vi "PROJECTE OCELL FINAL 0.3.vi"() -> ()   [LabVIEW 2020]
uses:
  <vilib>/numeric/Random Number (Range) DBL.vi
  <vilib>/MakerHub/LINX/Public/Utilities/Open Serial.vi
  <vilib>/MakerHub/LINX/LMH-LINX.lvlib
  <vilib>/MakerHub/LINX/Public/Sensors/Distance/Ultrasonic/Ultrasonic.lvlib
panel:
  in  "DO Channel 2":u8=11
  in  "DI Channel 2":u8=10
  out "Error Out 2":errorcluster
  in  "Sensibilitat 2":dbl=10.0
  in  "Sensibilitat 1":dbl=10.0
  in  "DO Channel 1":u8=6
  out "?":string="HEU GUANYAT !!!"
  in  "TEMPS D'ESPERA":i32=30
  in  "Velocitat de moviment":u32=100
  out "Error Out 1":errorcluster
  in  "?":bool
  in  "DI Channel 1":u8=5
  out "Device Name":string
  in  "Error In":errorcluster
  in  "Baud Rate Override":u32=9600
  in  "Serial Port":refnum<visa-resource-name>="COM3"
  out "JOC COL·LABORATIU: encertar l'ocell":cluster{dbl[], dbl[]}[](graph)=[{[0.99, 0.985, 0.98, 0.975, 0.86, 0.88, 0.9, 0.92, 0.94, 0.96, 0.98, 1.0, 0.94, 0.96, 0.98, 0.86], [41.0, 42.0, 43.0, 44.0, 45.0, 45.0, 45.0, 45.0, 45.0, 45.0, 45.0, 45.0, 44.0, 43.0, 42.0, 45.5]}, {[0.0, 0.0, 0.0, 0.02, 0.02, 0.02, 0.04, 0.04, 0.06, -0.06, -0.04, -0.04, -0.02, -0.02, -0.02], [43.0, 45.0, 44.0, 45.0, 46.0, 44.0, 46.0, 47.0, 47.0, 47.0, 47.0, 46.0, 46.0, 44.0, 45.0]}, {[-0.99, -0.985, -0.98, -0.975, -0.86, -0.88, -0.9, -0.92, -0.94, -0.96, -0.98, -1.0, -0.94, -0.96, -0.98, -0.86], [41.0, 42.0, 43.0, 44.0, 45.0, 45.0, 45.0, 45.0, 45.0, 45.0, 45.0, 45.0, 44.0, 43.0, 42.0, 45.5]}]
  # "CONTROLS\nARDUINO"
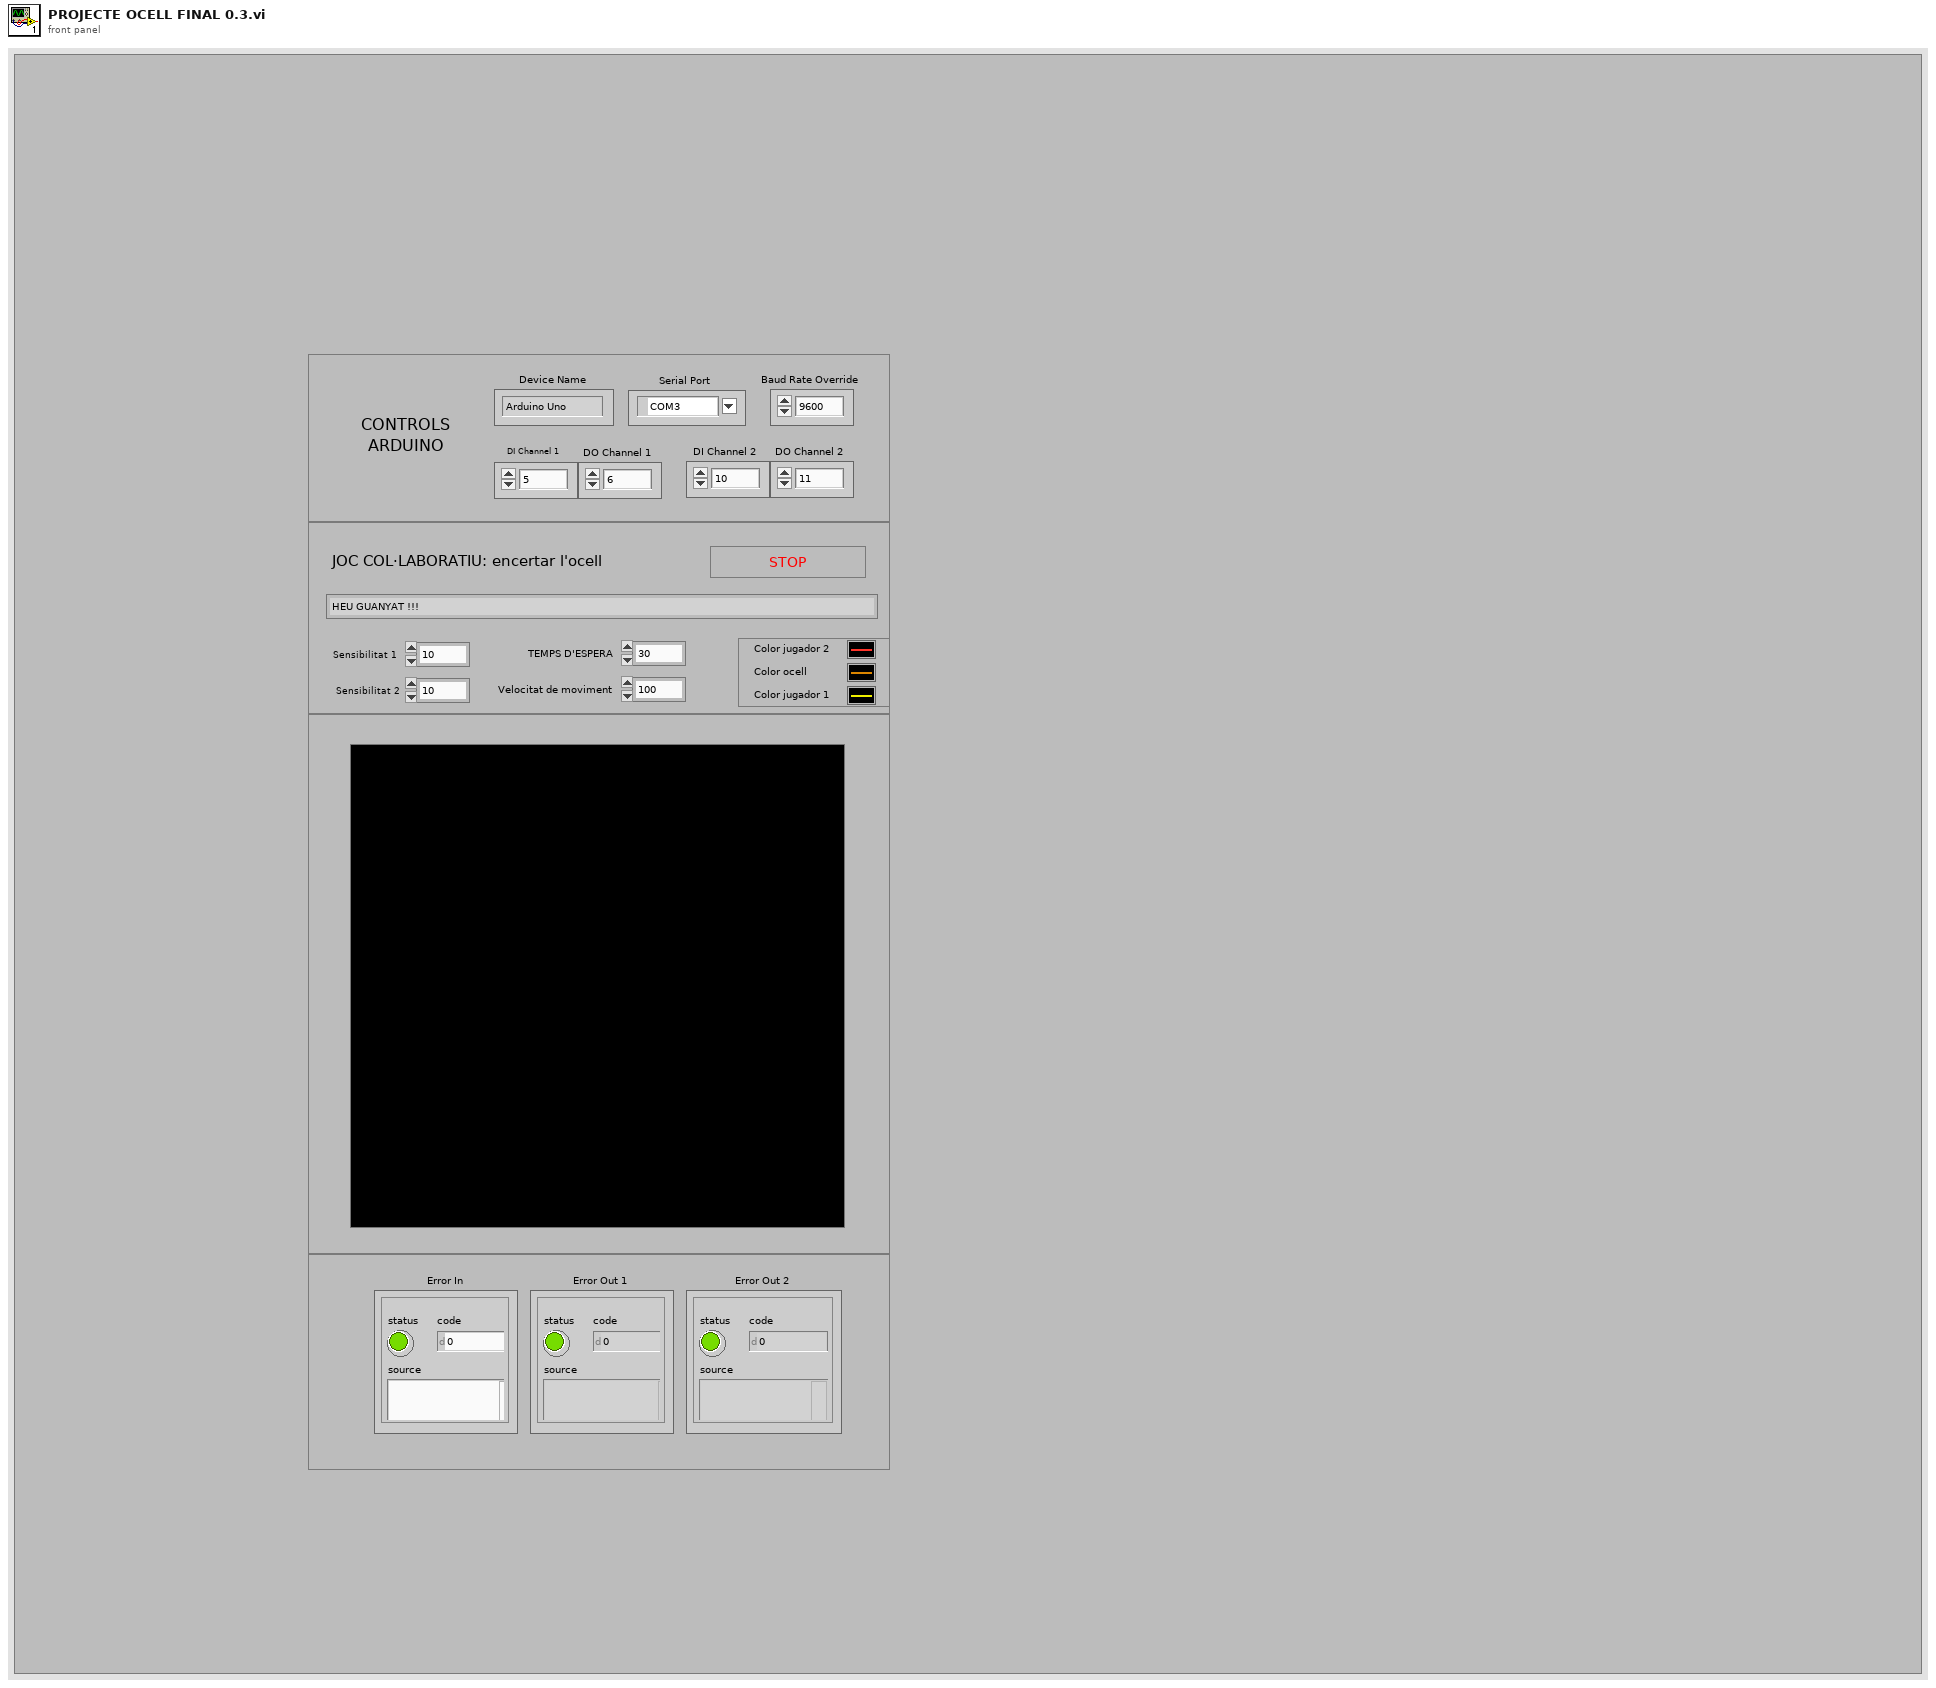
[diagram p1: front panel]
types:
  T1 = typedef "LMH-LINX.lvlib/LINX Ref.ctl" = cluster{"IO":T2, "Interface":T3, "LINX Device Config":T4}
  T2 = typedef "LMH-LINX.lvlib/Platform.ctl" = enum16{"Remote", "Local"}
  T3 = typedef "LMH-LINX.lvlib/Interface.ctl" = enum16{"Serial", "TCP"}
  T4 = typedef "LMH-LINX.lvlib/Device.lvlib/LINX Device Config.ctl" = cluster{"Interface":T3, "COM Port":refnum<visa-resource-name>, "TCP Configuration":T5, "Device Family":u8, "Device ID":u8, "Device Name":string, "TCP Ref":refnum<k5>, "Channels":T6}
  T5 = typedef "LMH-LINX.lvlib/Device.lvlib/TCP Config.ctl" = cluster{"IP Address":string, "Port":u16}
  T6 = typedef "LMH-LINX.lvlib/Channels.ctl" = cluster{"DI":u8[], "DO":u8[], "AI":u8[], "AO":u8[], "PWM":u8[], "QE":u8[], "UART":u8[], "I2C 2":u8[], "SPI":u8[], "CAN":u8[], "Servo":u8[], "AI Ref (V)":dbl, "AI Resolution (Bits)":u8, "AO Ref (V)":dbl, "AO Resolution (Bits)":u8}
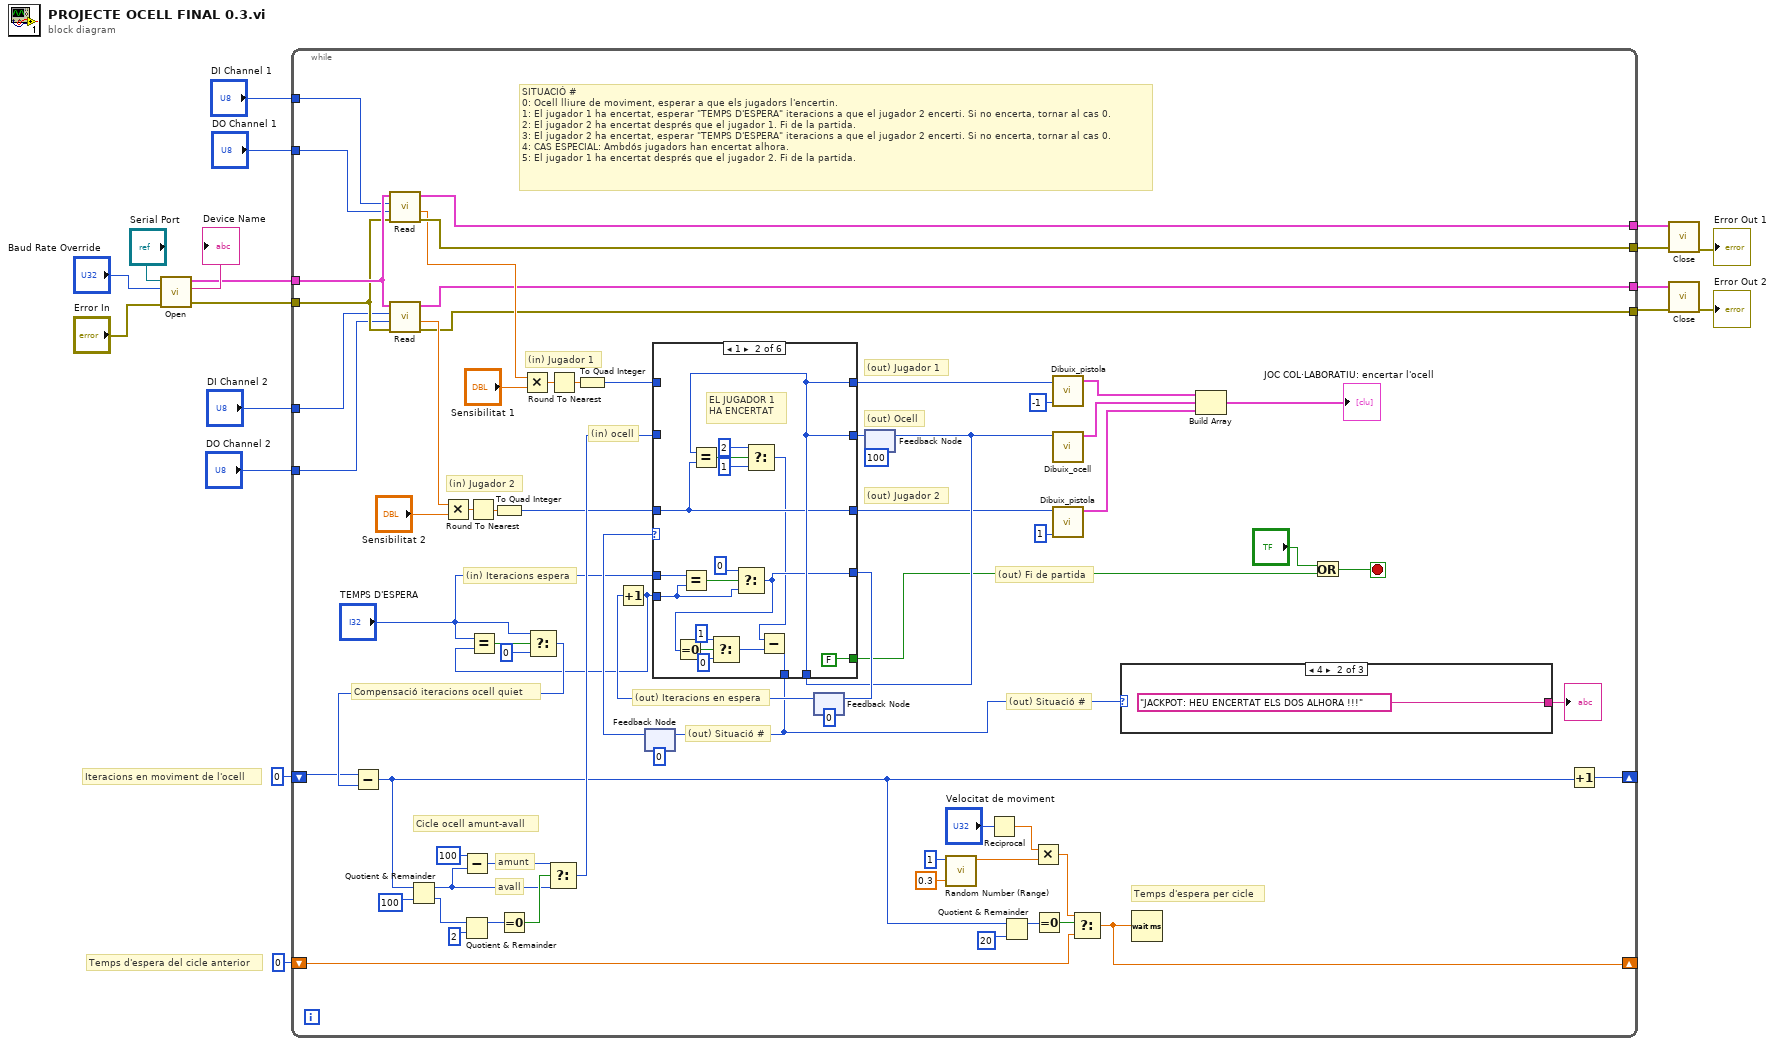
[diagram p0: block diagram]
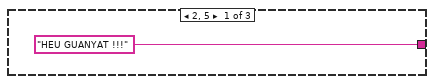
[diagram p2: hidden frame]
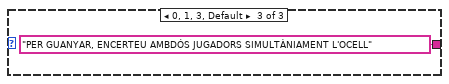
[diagram p3: hidden frame]
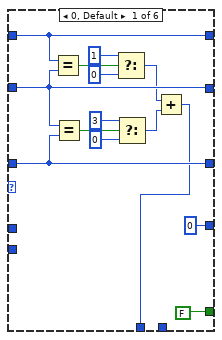
[diagram p4: hidden frame]
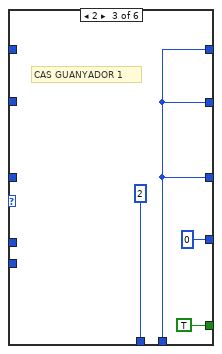
[diagram p5: hidden frame]
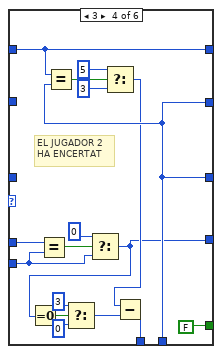
[diagram p6: hidden frame]
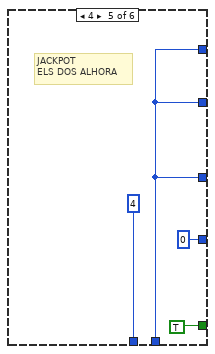
[diagram p7: hidden frame]
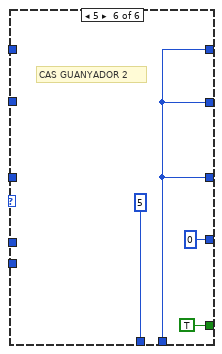
[diagram p8: hidden frame]
diagram:
  # "Temps d'espera del cicle anterior"
  # "Iteracions en moviment de l'ocell"
  n1 = call-poly <vilib>:"Open.vi"("Error In"="Error In", "Baud Rate Override"="Baud Rate Override", "Serial Port"="Serial Port") -> ("Error Out"=w14:errorcluster, "Device Name"=→"Device Name":string, "LINX Resource"=w15:T1)  [unwired: 6 in]
  n2 = while {
    tunnel: w15 -> [w38]
    tunnel: w14 -> [w36]
    tunnel: [w86] -> w13
    tunnel: [w85] -> w12
    shift-right: [w65] -> _
    shift-left: 0 -> [w63]
    shift-right: [w51] -> _
    shift-left: 0 -> [w52]
    tunnel: [w35] -> w8
    tunnel: [w34] -> w7
    tunnel: "DO Channel 1" -> [w28]
    tunnel: "DI Channel 1" -> [w27]
    tunnel: "DO Channel 2" -> [w26]
    tunnel: "DI Channel 2" -> [w25]
    stop <- w72 stop-if-true
    # "(out) Iteracions en espera"
    # "(in) Iteracions espera"
    # "(out) Situació #"
    # "(out) Fi de partida"
    # "SITUACIÓ #\n0: Ocell lliure de moviment, esperar a que els jugadors l'encertin.\n1: El jugador 1 ha encertat, esperar \"TEMPS D'ESPERA\" iteracions a que el jugador 2 encerti. Si no encerta, tornar al cas 0.\n2: El jugador 2 ha encertat després que el jugador 1. Fi de la partida.\n3: El jugador 2 ha encertat, esperar \"TEMPS D'ESPERA\" iteracions a que el jugador 2 encerti. Si no encerta, tornar al cas 0.\n4: CAS ESPECIAL: Ambdós jugadors han encertat alhora.\n5: El jugador 1 ha encertat després que el jugador 2. Fi de la partida."
    # "(out) Situació #"
    # "(in) ocell"
    # "avall"
    # "amunt"
    # "Temps d'espera per cicle"
    # "Compensació iteracions ocell quiet"
    # "(in) Jugador 2"
    # "(in) Jugador 1"
    # "Cicle ocell amunt-avall"
    # "(out) Jugador 2"
    # "(out) Jugador 1"
    # "(out) Ocell"
    n3 = call <vilib>:"Read.vi"("Error In"=w36, "DO Channel"=w28, "DI Channel"=w27, "LINX Resource"=w38) -> ("Error Out"=w85:errorcluster, "Centimeters"=w40:dbl, "LINX Resource"=w86:T1)  [unwired: 4 in, 1 out]
    n4 = call <vilib>:"Read.vi"("Error In"=w36, "DO Channel"=w26, "DI Channel"=w25, "LINX Resource"=w38) -> ("Error Out"=w34:errorcluster, "Centimeters"=w39:dbl, "LINX Resource"=w35:T1)  [unwired: 4 in, 1 out]
    n5 = Multiply(x=w39, y="Sensibilitat 2") -> (x*y=w37:dbl)
    n6 = Round To Nearest(number=w37) -> (nearest integer value=w77:dbl)
    n7 = To Quad Integer(1:w77) -> (0:w30:i64)
    n8 = Multiply(x=w40, y="Sensibilitat 1") -> (x*y=w43:dbl)
    n9 = Round To Nearest(number=w43) -> (nearest integer value=w41:dbl)
    n10 = To Quad Integer(1:w41) -> (0:w32:i64)
    n11 = feedback #1(0 ("f")) -> (w74:i32)
    n12 = feedback #2(0 ("t")) -> (w66:i32)
    n13 = Increment(x=w66) -> (x+1=w61:i32)
    n14 = Equal?(x="TEMPS D'ESPERA", y=w61) -> (x = y?=w68:bool)
    n15 = Select(t="TEMPS D'ESPERA", s=w68, f=0) -> (s? t:f=w64:i32)
    n16 = Subtract(x=w63, y=w64) -> (x-y=w59:i32)
    n17 = Quotient & Remainder(x=w59, y=100) -> (x-y*floor(x/y)=w19:i32, floor(x/y)=w80:i32)
    n18 = Subtract(x=100 ("y"), y=w19) -> (x-y=w82:i32)
    n19 = Quotient & Remainder(x=w80, y=2) -> (x-y*floor(x/y)=w78:i32)  [unwired: 1 out]
    n20 = Equal To 0?(x=w78) -> (x = 0?=w79:bool)
    n21 = Select(t=w82, s=w79, f=w19) -> (s? t:f=w69:i32)
    n22 = feedback #3(100) -> (w47:i32)
    n23 = case shown="1" w74 {
      tunnel: w32 -> [w104 _ _ w139 _ _]
      tunnel: [w104 w118 w124 w139 w145 w149] -> w31
      tunnel: w69 -> [w97 _ _ _ _ _]
      tunnel: [w97 w118 w124 w138 w145 w149] -> w76
      tunnel: w47 -> [_ w118 w124 w138 w145 w149]
      tunnel: w30 -> [w96 w117 _ _ _ _]
      tunnel: [w96 w117 w124 w138 w145 w149] -> w29
      tunnel: [w93 w109 2 ("f") w129 4 ("f") 5 ("f")] -> w45
      tunnel: w61 -> [_ w113 _ w128 _ _]
      tunnel: [0 ("t") w111 0 ("t") w126 0 ("t") 0 ("t")] -> w71
      tunnel: "TEMPS D'ESPERA" -> [_ w112 _ w127 _ _]
      tunnel: [FALSE FALSE TRUE FALSE TRUE TRUE] -> w23
      frame 0, Default {
        n24 = Equal?(x=w104, y=w97) -> (x = y?=w103:bool)
        n25 = Equal?(x=w97, y=w96) -> (x = y?=w100:bool)
        n26 = Select(t=1, s=w103, f=0) -> (s? t:f=w94:i32)
        n27 = Select(t=3, s=w100, f=0) -> (s? t:f=w95:i32)
        n28 = Add(x=w94, y=w95) -> (x+y=w93:i32)
      }
      frame 1 {
        # "EL JUGADOR 1\nHA ENCERTAT"
        n29 = Equal?(x=w112, y=w113) -> (x = y?=w115:bool)
        n30 = Equal?(x=w118, y=w117) -> (x = y?=w121:bool)
        n31 = Select(t=0, s=w115, f=w113) -> (s? t:f=w111:i32)
        n32 = Equal To 0?(x=w111) -> (x = 0?=w107:bool)
        n33 = Select(t=1, s=w107, f=0 ("t")) -> (s? t:f=w108:i32)
        n34 = Select(t=2, s=w121, f=1) -> (s? t:f=w110:i32)
        n35 = Subtract(x=w110, y=w108) -> (x-y=w109:i32)
      }
      frame 2 {
        # "CAS GUANYADOR 1"
      }
      frame 3 {
        # "EL JUGADOR 2\nHA ENCERTAT"
        n36 = Equal?(x=w127, y=w128) -> (x = y?=w136:bool)
        n37 = Equal?(x=w139, y=w138) -> (x = y?=w142:bool)
        n38 = Select(t=0, s=w136, f=w128) -> (s? t:f=w126:i32)
        n39 = Equal To 0?(x=w126) -> (x = 0?=w133:bool)
        n40 = Select(t=3, s=w133, f=0 ("t")) -> (s? t:f=w134:i32)
        n41 = Select(t=5, s=w142, f=3) -> (s? t:f=w130:i32)
        n42 = Subtract(x=w130, y=w134) -> (x-y=w129:i32)
      }
      frame 4 {
        # "JACKPOT\nELS DOS ALHORA"
      }
      frame 5 {
        # "CAS GUANYADOR 2"
      }
    }
    n43 = feedback-in #1(w45) -> ()
    n44 = feedback-in #2(w71) -> ()
    n45 = feedback-in #3(w76) -> ()
    n46 = call-poly <vilib>:"Random Number (Range).vi"("lower bound (0)"=0.3, "upper bound (100)"=u64 1) -> ("number"=w54:dbl)  [unwired: 9 in]
    n47 = Reciprocal(x="Velocitat de moviment") -> (1/x=w20:dbl)
    n48 = Quotient & Remainder(x=w59, y=20 ("f")) -> (x-y*floor(x/y)=w58:i32)  [unwired: 1 out]
    n49 = Multiply(x=w20, y=w54) -> (x*y=w53:dbl)
    n50 = Equal To 0?(x=w58) -> (x = 0?=w57:bool)
    n51 = call "Dibuix_pistola.vi"("Esquerra/Dreta (-1/1)"=-1, "Posició Y"=w31) -> ("Dibuix pistola"=w22:cluster{dbl[], dbl[]})  [unwired: 9 in]
    n52 = call "Dibuix_ocell.vi"("Posició Y"=w47) -> ("Dibuix pistola"=w46:cluster{dbl[], dbl[]})  [unwired: 10 in]
    n53 = call "Dibuix_pistola.vi"("Esquerra/Dreta (-1/1)"=1, "Posició Y"=w29) -> ("Dibuix pistola"=w49:cluster{dbl[], dbl[]})  [unwired: 9 in]
    n54 = Select(t=w53, s=w57, f=w52) -> (s? t:f=w51:dbl)
    n55 = case shown="4" w45 {
      tunnel: ["HEU GUANYAT !!!" "JACKPOT: HEU ENCERTAT ELS DOS ALHORA !!!" "PER GUANYAR, ENCERTEU AMBDÓS JUGADORS SIMULTÀNIAMENT L'OCELL"] -> w44
      frame 2, 5 {
      }
      frame 4 {
      }
      frame 0, 1, 3, Default {
      }
    }
    "?" <- w44
    n56 = Wait (ms)(milliseconds to wait=w51) -> ()  [unwired: 1 out]
    n57 = Build Array(w22, w46, w49) -> (→"JOC COL·LABORATIU: encertar l'ocell":cluster{dbl[], dbl[]}[])
    n58 = Or(x="?", y=w23) -> (x .or. y?=w72:bool)
    n59 = Increment(x=w59) -> (x+1=w65:i32)
  }
  n60 = call <vilib>:"Close.vi"("Error In"=w12, "LINX Resource"=w13) -> ("Error Out"=→"Error Out 1":errorcluster)  [unwired: 9 in]
  n61 = call <vilib>:"Close.vi"("Error In"=w7, "LINX Resource"=w8) -> ("Error Out"=→"Error Out 2":errorcluster)  [unwired: 9 in]
